vi "Units_RotationsToRadians.vi"(10 "Rotations":dbl) -> (2 "Radians":dbl)   [LabVIEW 2019, in "Trajectory_Library.lvlib"]
doc: "Convert a value from rotations to radians\n\nInputs: \n - Rotations - Angle (rotations)\n\nOutputs:\n - Radians - Angle (Radians)"
uses:
  Trajectory_Library.lvlib
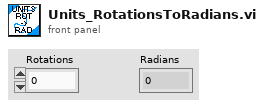
[diagram p1: front panel]
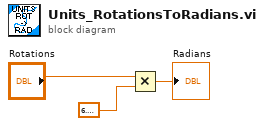
[diagram p0: block diagram]
diagram:
  n1 = Multiply(x="Rotations", y=6.283185307179586) -> (x*y=→"Radians":dbl)
